vi "Service ID.vi"(8 "error in (no error)":errorcluster, 11 "User Provider in":refnum<class "User Provider.lvclass">) -> (0 "error out":errorcluster, 2 "Service ID":string, 3 "User Provider out":refnum<class "User Provider.lvclass">)   [LabVIEW 2020, in "HTTP Server.lvlib" / "User Provider.lvclass"]
uses:
  User Provider.lvclass
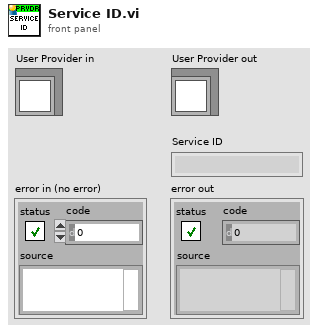
[diagram p1: front panel]
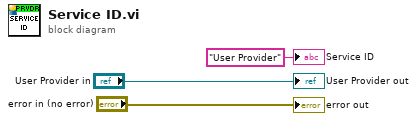
[diagram p0: block diagram]
diagram:
  "error out" <- "error in (no error)"
  "User Provider out" <- "User Provider in"
  "Service ID" <- "User Provider" ("Service ID")
